vi "Get Software Details.vi"(6 "Trace Component Info (F)":bool, 8 "error in (no error)":errorcluster, 11 "Enumerator in":u64) -> (0 "error out":errorcluster, 3 "Software Component":T1 {"component type" items=["standard", "hidden", "system", "unknown", "startup", "image", "essential"]})   [LabVIEW 2020, in "nisyscfg.lvlib"]
uses:
  <vilib>/nisyscfg/nisyscfg.lvlib
  <vilib>/nisyscfg/Software 1.2.ctl
  <vilib>/nisyscfg/Component Type.ctl
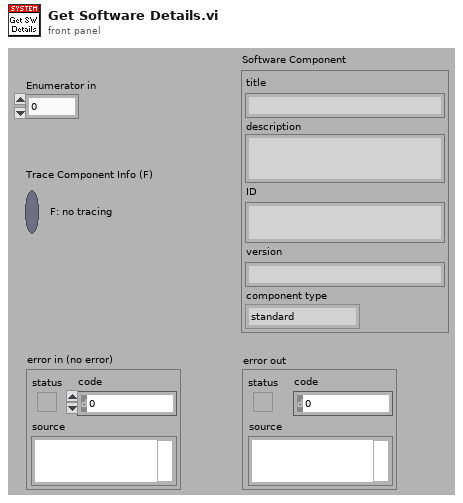
[diagram p1: front panel]
types:
  T1 = typedef "nisyscfg.lvlib/Software 1.2.ctl" = cluster{"title":string, "description":string, "ID":string, "version":string, "component type":T2}
  T2 = typedef "nisyscfg.lvlib/Component Type.ctl" = u32
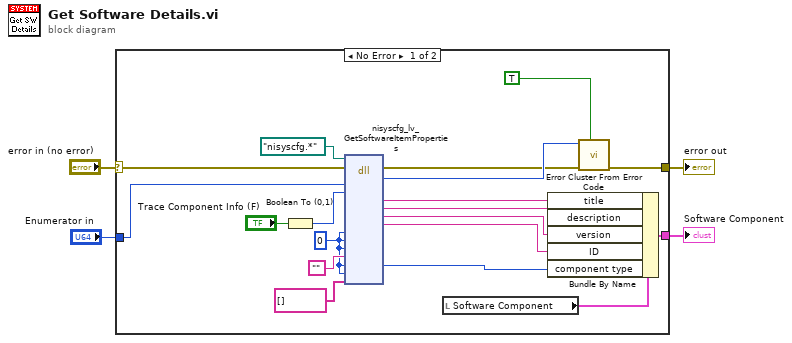
[diagram p0: block diagram]
diagram:
  n1 = case shown="No Error" "error in (no error)" {
    selector: "error in (no error)" -> [w15 w24]
    tunnel: [w12 w24] -> w3
    tunnel: [w13 _] -> w1
    tunnel: "Enumerator in" -> [w14 _]
    frame No Error {
      w16 = u32 0 ("isAvailable")
      n2 = Boolean To (0,1)(Boolean="Trace Component Info (F)") -> (0, 1=w10:i16)
      n3 = dll-call lib="nisyscfg.*" fn="nisyscfg_lv_GetSoftwareItemProperties" label="GetSoftwareItemProperties"(path in=path "nisyscfg.*", error in=w15, "item"=w14, "logToSpy"=w10, "hideVersion"=w16, "numChildren"=w16, "type"=w16, "oldestCompatibleVersion"="", "visibilityType"=w16, "isAvailable"=w16, "childrenIDs"=string[] [] ("Array")) -> (error out=w22:errorcluster, "result"=w23:i32, "title"=w6:string, "description"=w7:string, "version"=w8:string, "ID"=w9:string, "visibilityType"=w5:u32)  [unwired: 13 in, 1 out]
      n4 = local read "Software Component"() -> (w17:T1)
      n5 = Bundle By Name(cluster=w17, "title"=w6, "description"=w7, "version"=w8, "ID"=w9, "component type"=w5) -> (w13:T1)
      n6 = call <vilib>:"Error Cluster From Error Code.vi"("show call chain? (False)"=TRUE, "error in (no error)"=w22, "error code (0)"=w23) -> ("error out"=w12:errorcluster)  [unwired: 6 in]
    }
    frame Error {
    }
  }
  "error out" <- w3
  "Software Component" <- w1
